vi "LCDGetWidth.vi"(8 "error in (no error)":errorcluster, 11 "Device In":u64) -> (0 "error out":errorcluster, 2 "Width":i32, 3 "Device Out":u64)   [LabVIEW 2012, in "Phidget LCD.lvlib"]
doc: "${Width:Header}"
uses:
  <instrlib>/Phidgets/Phidget LCD/Phidget LCD.lvlib
  <instrlib>/Phidgets/Phidget Common/Phidget Common.lvlib
  phidget22.dll
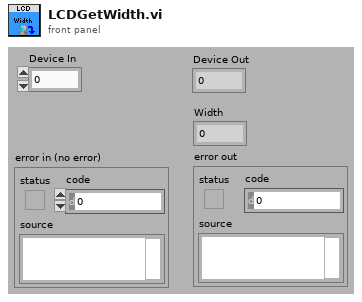
[diagram p1: front panel]
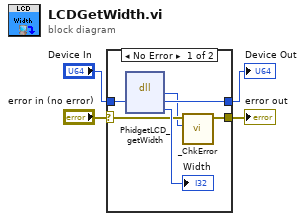
[diagram p0: block diagram]
diagram:
  n1 = case shown="No Error" "error in (no error)" {
    selector: "error in (no error)" -> [w7 w12]
    tunnel: [w6 w12] -> w3
    tunnel: "Device In" -> [w9 w11]
    tunnel: [w8 w11] -> w1
    frame No Error {
      n2 = dll-call lib="phidget22.*" fn="PhidgetLCD_getWidth"("phid"=w9) -> ("return type"=w5:i32, "phid"=w8:u64, "count"=→"Width":i32)  [unwired: 4 in, 2 out]
      n3 = call <instrlib>:"_ChkError.vi"("Return Code"=w5, "error in (no error)"=w7) -> ("error out"=w6:errorcluster)  [unwired: 9 in]
    }
    frame Error {
    }
  }
  "error out" <- w3
  "Device Out" <- w1
